vi "验证操作权限.vi"(9 "权限选择":u16(ring), 10 "密码":string) -> (2 "验证成功":bool)   [LabVIEW 2017]
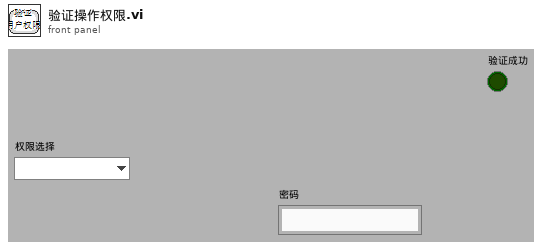
[diagram p1: front panel]
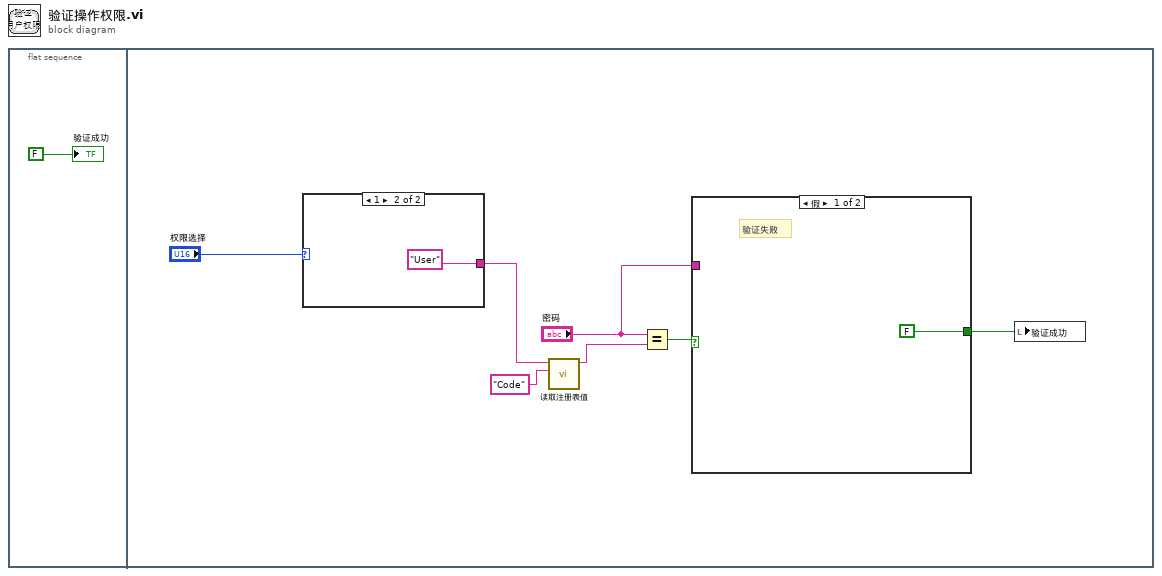
[diagram p0: block diagram]
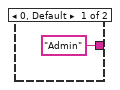
[diagram p2: hidden frame]
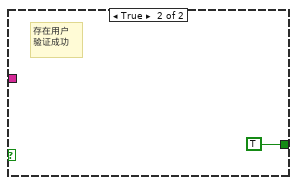
[diagram p3: hidden frame]
diagram:
  n1 = flat-sequence {
    frame #0 {
      "验证成功" <- FALSE ("验证成功")
    }
    frame #1 {
      n2 = case shown="1" "权限选择" {
        tunnel: ["Admin" ("subkeyName") "User" ("subkeyName")] -> w5
        frame 0, Default {
        }
        frame 1 {
        }
      }
      n3 = call "读取注册表值.vi"("value"="Code", "subkeyName"=w5) -> ("Data"=w3:string)  [unwired: 7 in]
      n4 = Equal?(x="密码", y=w3) -> (x = y?=w8:bool)
      n5 = case shown="假" w8 {
        tunnel: "密码" -> [_ _]
        tunnel: [FALSE TRUE] -> w6
        frame False {
          # "验证失败"
        }
        frame True {
          # "存在用户\n验证成功"
        }
      }
      n6 = local write "验证成功"(w6) -> ()
    }
  }
